vi "Get VI Name.vi"(8 "error in (no error)":errorcluster, 11 "VI Call In":refnum<class "VI Call.lvclass">) -> (0 "error out":errorcluster, 2 "VI Name":string)   [LabVIEW 2020, in "VI Call.lvclass"]
uses:
  VI Call.lvclass
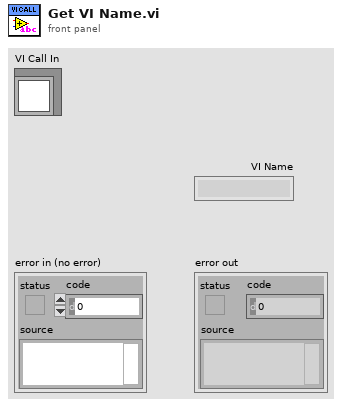
[diagram p1: front panel]
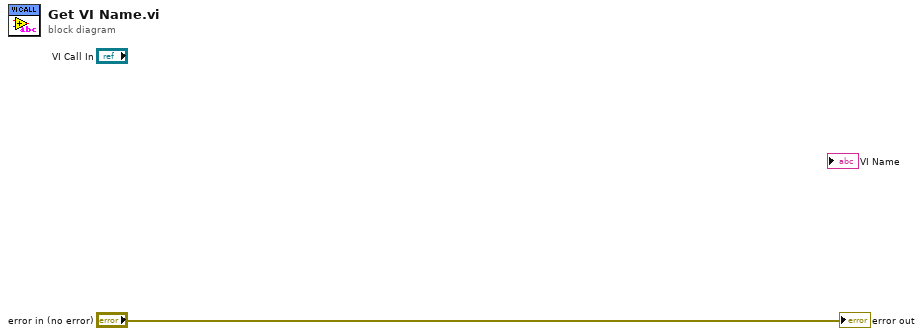
[diagram p0: block diagram]
diagram:
  "error out" <- "error in (no error)"
